vi "Json to Tokens.vi"(0 "JSON String":string, 11 "Error In":errorcluster) -> (4 "JSON Tokens":string[](array[string]), 15 "Error Out":errorcluster)   [LabVIEW 2019, in "JsonToCluster.lvlib"]
doc: "This VI converts JSON string into array of tokens"
uses:
  JsonToCluster.lvlib
  <vilib>/regexp/Match Regular Expression.xnode
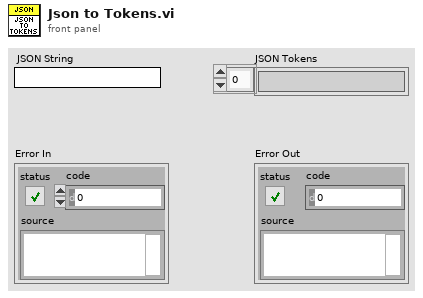
[diagram p1: front panel]
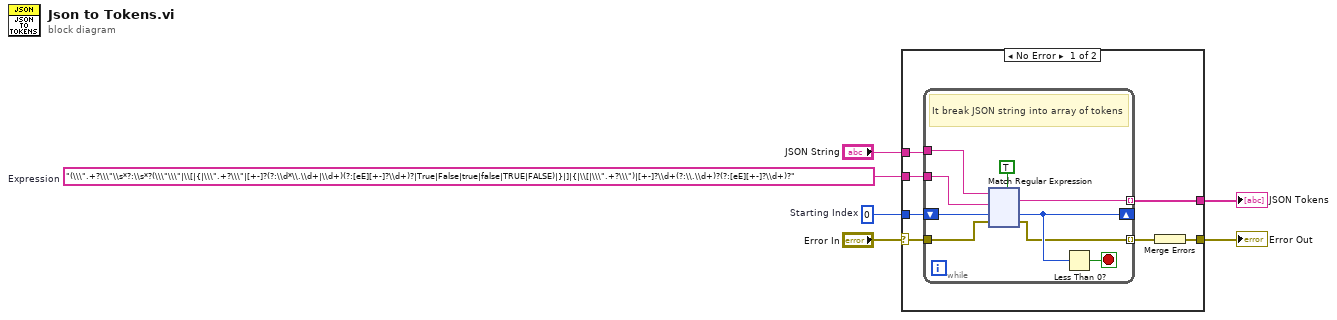
[diagram p0: block diagram]
diagram:
  w6 = "(\\\".+?\\\"\\s*?:\\s*?(\\\"\\\"|\\[|{|\\\".+?\\\"|[+-]?(?:\\d*\\.\\d+|\\d+)(?:[eE][+-]?\\d+)?|True|False|true|false|TRUE|FALSE)|}|]|{|\\[|\\\".+?\\\")|[+-]?\\d+(?:\\.\\d+)?(?:[eE][+-]?\\d+)?"  # Expression
  w3 = 0  # Starting Index
  n1 = case shown="No Error" "Error In" {
    selector: "Error In" -> [w9 w137]
    tunnel: w6 -> [w13 _]
    tunnel: [w12 _] -> w5
    tunnel: "JSON String" -> [w11 _]
    tunnel: w3 -> [w10 _]
    tunnel: [w7 w137] -> w1
    frame No Error {
      n2 = while {
        tunnel: w11 -> [w21]
        shift-right: [w17] -> _
        shift-left: w10 -> [w20]
        tunnel: [w19] -> w12 mode=indexing
        tunnel: w13 -> [w16]
        tunnel: [w15] -> w8 mode=indexing
        tunnel: w9 -> [w14]
        stop <- w22 stop-if-true
        # "It break JSON string into array of tokens"
        n3 = xnode "Match Regular Expression"("input string"=w21, "regular expression"=w16, "offset (0)"=w20, "error in"=w14, "multiline? (F)"=TRUE) -> ("whole match"=w19:string, "offset past match"=w17:i32, "error out"=w15:errorcluster)  [unwired: 1 in, 2 out]
        n4 = Less Than 0?(x=w17) -> (x < 0?=w22:bool)
      }
      n5 = Merge Errors(w8) -> (w7:errorcluster)
    }
    frame Error {
    }
  }
  "JSON Tokens" <- w5
  "Error Out" <- w1
